vi "HeatFlow Results File Init.vi"(8 "error in":errorcluster, 9 "HeatFlow Res Cfg":T1, 11 "Log File Base Path":path) -> (0 "error out":errorcluster, 1 "Log File Name":string, 3 "Refnum out":refnum<k34>)   [LabVIEW 2019, in "Logging.lvlib"]
uses:
  Logging.lvlib
  HeatFlow Results States.ctl
  HeatFlow Res Cfg.ctl
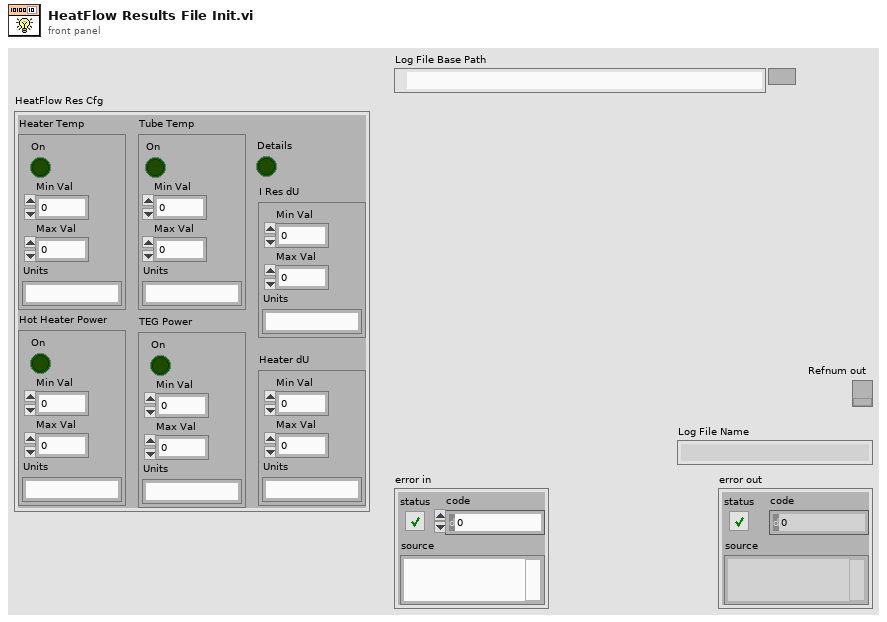
[diagram p1: front panel]
types:
  T1 = typedef "Logging.lvlib/HeatFlow Res Cfg.ctl" = cluster{"Heater Temp":cluster{"On":bool, "Min Val":dbl, "Max Val":dbl, "Units":string}, "Tube Temp":cluster{"On":bool, "Min Val":dbl, "Max Val":dbl, "Units":string}, "Hot Heater Power":cluster{"On":bool, "Min Val":dbl, "Max Val":dbl, "Units":string}, "TEG Power":cluster{"On":bool, "Min Val":dbl, "Max Val":dbl, "Units":string}, "Details":bool, "Heater dU":cluster{"Min Val":dbl, "Max Val":dbl, "Units":string}, "I Res dU":cluster{"Min Val":dbl, "Max Val":dbl, "Units":string}}
  T2 = typedef "Logging.lvlib/HeatFlow Results States.ctl" = enum16{"Start", "Timestamp", "Heater Temp", "Tube Temp", "Heater Power", "TEG Power", "Details", "End"}
  T3 = enum16{"open", "open or create", "create or replace", "create", "open (read-only)"}
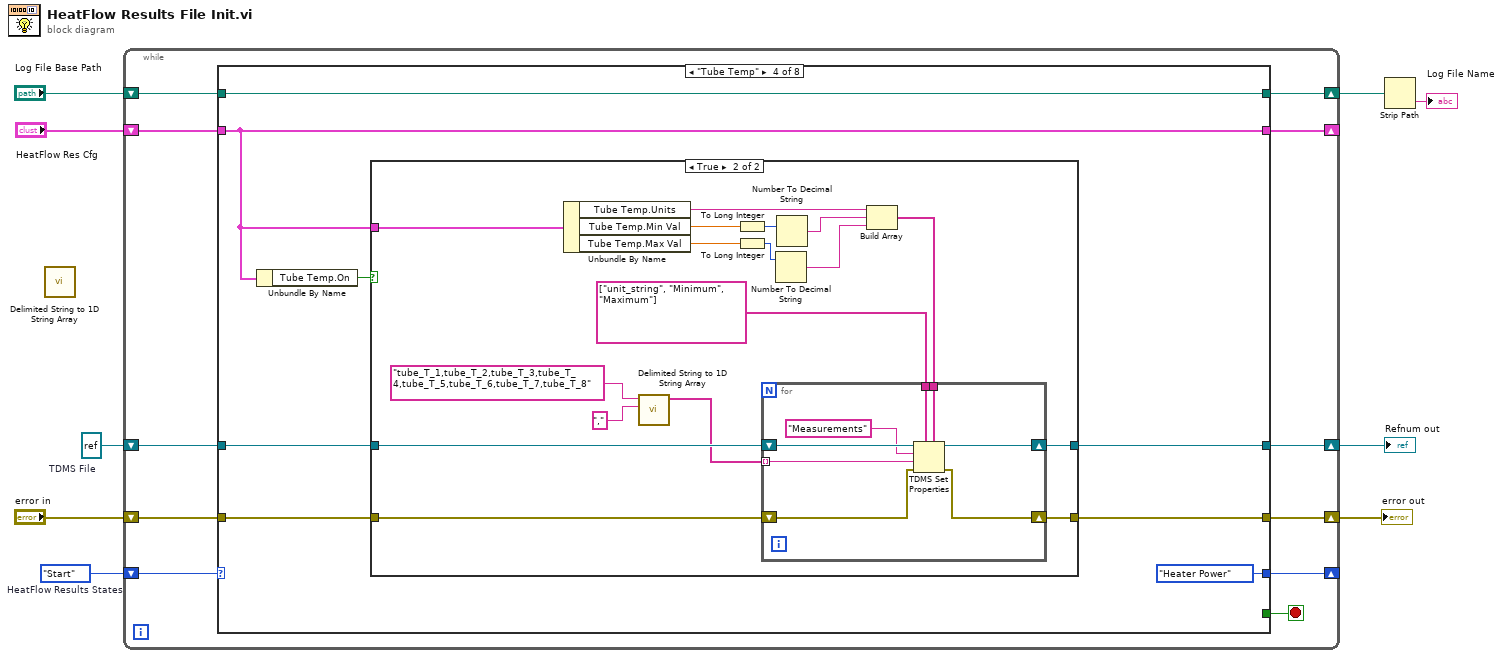
[diagram p0: block diagram]
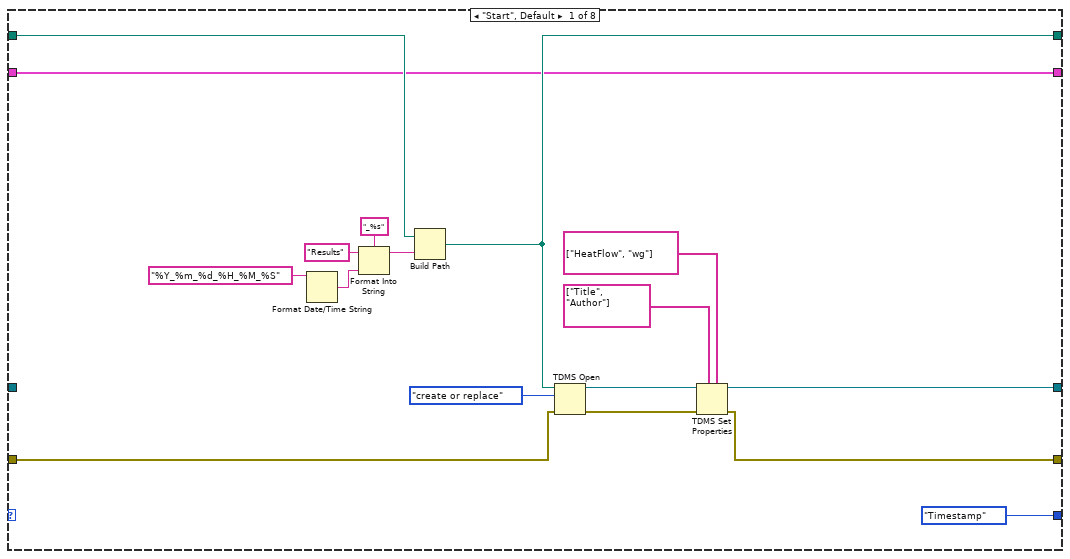
[diagram p2: hidden frame]
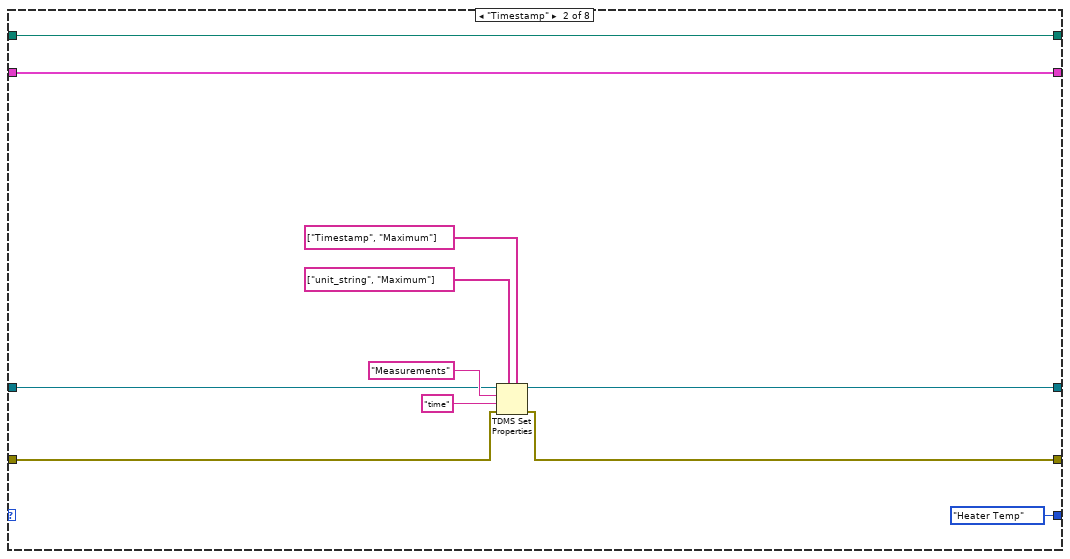
[diagram p3: hidden frame]
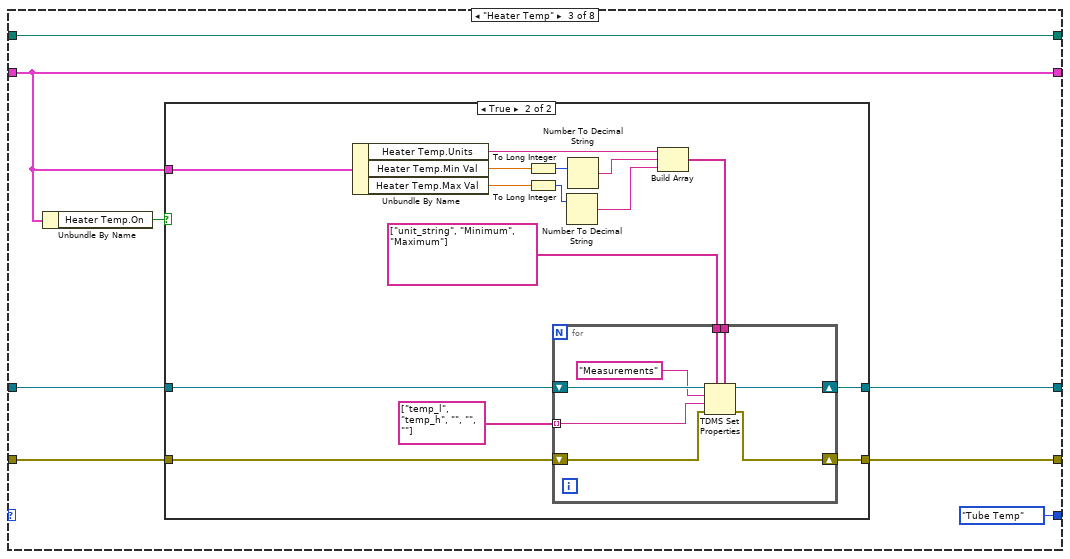
[diagram p4: hidden frame]
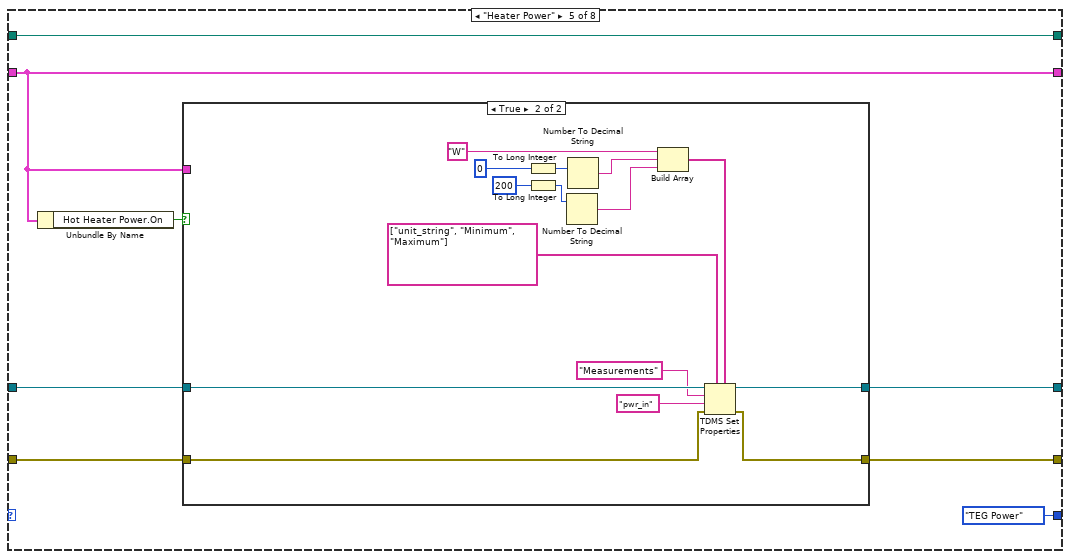
[diagram p7: hidden frame]
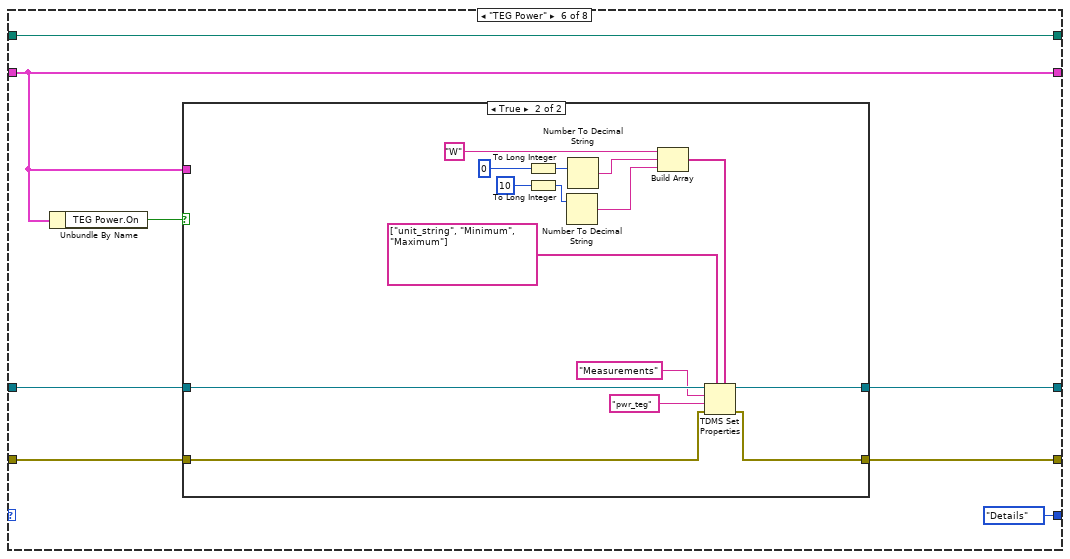
[diagram p9: hidden frame]
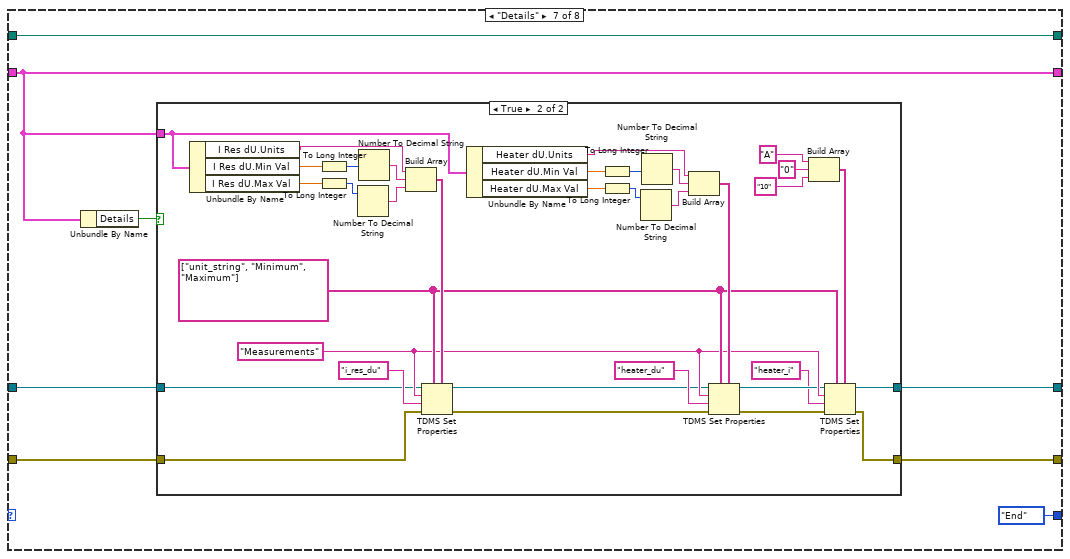
[diagram p11: hidden frame]
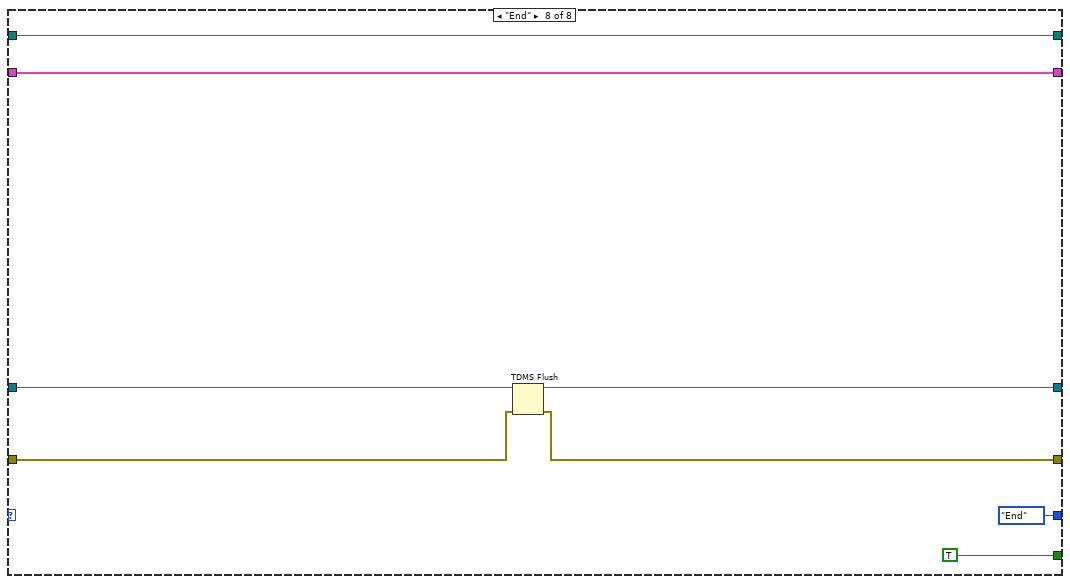
[diagram p13: hidden frame]
diagram:
  w2 = HeatFlow_Results_States."Start"  # HeatFlow Results States
  w8 = refnum<k34> refnum  # TDMS File
  n1 = call <vilib>:"Delimited String to 1D String Array.vi"() -> ()  [unwired: 11 in, 1 out]
  n2 = while {
    shift-right: [w10] -> _
    shift-left: w2 -> [w13]
    shift-right: [w17] -> w4
    shift-left: "Log File Base Path" -> [w20]
    shift-right: [w18] -> w7
    shift-left: "error in" -> [w19]
    shift-right: [w11] -> _
    shift-left: "HeatFlow Res Cfg" -> [w12]
    shift-right: [w15] -> w5
    shift-left: w8 -> [w16]
    stop <- w14 stop-if-true
    n3 = case shown="\"Tube Temp\"" w13 {
      tunnel: w20 -> [w31 w42 w56 w89 w124 w149 w173 w218]
      tunnel: w19 -> [w24 w41 w53 w86 w121 w146 w170 w214]
      tunnel: [w23 w40 w52 w85 w120 w145 w168 w213] -> w18
      tunnel: [w30 w42 w56 w89 w124 w149 w173 w218] -> w17
      tunnel: w16 -> [_ w44 w55 w88 w123 w148 w171 w216]
      tunnel: [w25 w43 w54 w87 w122 w147 w169 w215] -> w15
      tunnel: [_ _ _ _ _ _ _ TRUE] -> w14
      tunnel: w12 -> [w22 w39 w49 w82 w117 w142 w167 w212]
      tunnel: [w22 w39 w49 w82 w117 w142 w167 w212] -> w11
      tunnel: [HeatFlow_Results_States."Timestamp" ("Results") HeatFlow_Results_States."Heater Temp" ("Results") HeatFlow_Results_States."Tube Temp" ("Results") HeatFlow_Results_States."Heater Power" ("Results") HeatFlow_Results_States."TEG Power" ("Results") HeatFlow_Results_States."Details" ("Results") HeatFlow_Results_States."End" ("Results") HeatFlow_Results_States."End" ("Results")] -> w10
      frame "Start", Default {
        n4 = Format Date/Time String(time format string (%c)="%Y_%m_%d_%H_%M_%S") -> (date/time string=w37:string)  [unwired: 2 in]
        n5 = Format Into String(format string="_%s", initial string="Results", w37) -> (resulting string=w36:string)  [unwired: 1 in, 1 out]
        n6 = Build Path(base path=w31, name or relative path=w36) -> (appended path=w30:path)
        n7 = TDMS Open(8:w24, 10:T3."create or replace" ("operation (0:open)"), 11:w30) -> (0:w28:errorcluster, 3:w29:refnum<k34>)  [unwired: 4 in]
        n8 = TDMS Set Properties(5:string[] ["HeatFlow", "wg"] ("property names"), 7:string[] ["Title", "Author"] ("property names"), 8:w28, 11:w29) -> (0:w23:errorcluster, 3:w25:refnum<k34>)  [unwired: 2 in, 2 out]
      }
      frame "Timestamp" {
        n9 = TDMS Set Properties(5:string[] ["Timestamp", "Maximum"] ("property names"), 7:string[] ["unit_string", "Maximum"] ("property names"), 8:w41, 9:"time" ("channel name"), 10:"Measurements" ("group name in (Untitled)"), 11:w44) -> (0:w40:errorcluster, 3:w43:refnum<k34>)  [unwired: 2 out]
      }
      frame "Heater Temp" {
        n10 = Unbundle By Name(w49) -> ("Heater Temp.On"=w51:bool)
        n11 = case shown="True" w51 {
          tunnel: w55 -> [w58 w73]
          tunnel: [w58 w72] -> w54
          tunnel: w53 -> [w57 w71]
          tunnel: [w57 w70] -> w52
          tunnel: w49 -> [_ w62]
          frame False {
          }
          frame True {
            n12 = Unbundle By Name(w62) -> ("Heater Temp.Units"=w61:string, "Heater Temp.Min Val"=w60:dbl, "Heater Temp.Max Val"=w59:dbl)
            n13 = To Long Integer(number=w60) -> (32bit integer=w66:i32)
            n14 = To Long Integer(number=w59) -> (32bit integer=w65:i32)
            n15 = Number To Decimal String(number=w65) -> (decimal integer string=w63:string)  [unwired: 1 in]
            n16 = Number To Decimal String(number=w66) -> (decimal integer string=w64:string)  [unwired: 1 in]
            n17 = Build Array(w61, w64, w63) -> (w67:string[])
            n18 = for {
              shift-right: [w80] -> w72
              shift-left: w73 -> [w81]
              shift-right: [w77] -> w70
              shift-left: w71 -> [w78]
              tunnel: string[] ["temp_l", "temp_h", "", "", ""] -> [w76] mode=indexing
              tunnel: string[] ["unit_string", "Minimum", "Maximum"] ("property names") -> [w75]
              tunnel: w67 -> [w74]
              n19 = TDMS Set Properties(5:w74, 7:w75, 8:w78, 9:w76, 10:"Measurements" ("group name in (Untitled)"), 11:w81) -> (0:w77:errorcluster, 3:w80:refnum<k34>)  [unwired: 2 out]
            }
          }
        }
      }
      frame "Tube Temp" {
        n20 = Unbundle By Name(w82) -> ("Tube Temp.On"=w84:bool)
        n21 = case shown="True" w84 {
          tunnel: w88 -> [w91 w108]
          tunnel: [w91 w107] -> w87
          tunnel: w86 -> [w90 w106]
          tunnel: [w90 w105] -> w85
          tunnel: w82 -> [_ w95]
          frame False {
          }
          frame True {
            n22 = Unbundle By Name(w95) -> ("Tube Temp.Units"=w94:string, "Tube Temp.Min Val"=w93:dbl, "Tube Temp.Max Val"=w92:dbl)
            n23 = call <vilib>:"Delimited String to 1D String Array.vi"("delimiter"=",", "delimited string"="tube_T_1,tube_T_2,tube_T_3,tube_T_4,tube_T_5,tube_T_6,tube_T_7,tube_T_8" ("name to assign")) -> ("string array"=w97:string[])  [unwired: 9 in]
            n24 = To Long Integer(number=w93) -> (32bit integer=w102:i32)
            n25 = To Long Integer(number=w92) -> (32bit integer=w101:i32)
            n26 = Number To Decimal String(number=w101) -> (decimal integer string=w99:string)  [unwired: 1 in]
            n27 = Number To Decimal String(number=w102) -> (decimal integer string=w100:string)  [unwired: 1 in]
            n28 = Build Array(w94, w100, w99) -> (w103:string[])
            n29 = for {
              shift-right: [w115] -> w107
              shift-left: w108 -> [w116]
              shift-right: [w112] -> w105
              shift-left: w106 -> [w113]
              tunnel: w97 -> [w111] mode=indexing
              tunnel: string[] ["unit_string", "Minimum", "Maximum"] ("property names") -> [w110]
              tunnel: w103 -> [w109]
              n30 = TDMS Set Properties(5:w109, 7:w110, 8:w113, 9:w111, 10:"Measurements" ("group name in (Untitled)"), 11:w116) -> (0:w112:errorcluster, 3:w115:refnum<k34>)  [unwired: 2 out]
            }
          }
        }
      }
      frame "Heater Power" {
        n31 = Unbundle By Name(w117) -> ("Hot Heater Power.On"=w119:bool)
        n32 = case shown="True" w119 {
          tunnel: w123 -> [w126 w141]
          tunnel: [w126 w140] -> w122
          tunnel: w121 -> [w125 w139]
          tunnel: [w125 w138] -> w120
          tunnel: w117 -> [_ _]
          frame False {
          }
          frame True {
            n33 = To Long Integer(number=0) -> (32bit integer=w135:i32)
            n34 = To Long Integer(number=200) -> (32bit integer=w134:i32)
            n35 = Number To Decimal String(number=w134) -> (decimal integer string=w132:string)  [unwired: 1 in]
            n36 = Number To Decimal String(number=w135) -> (decimal integer string=w133:string)  [unwired: 1 in]
            n37 = Build Array("W" ("element"), w133, w132) -> (w136:string[])
            n38 = TDMS Set Properties(5:w136, 7:string[] ["unit_string", "Minimum", "Maximum"] ("property names"), 8:w139, 9:"pwr_in" ("channel name"), 10:"Measurements" ("group name in (Untitled)"), 11:w141) -> (0:w138:errorcluster, 3:w140:refnum<k34>)  [unwired: 2 out]
          }
        }
      }
      frame "TEG Power" {
        n39 = Unbundle By Name(w142) -> ("TEG Power.On"=w144:bool)
        n40 = case shown="True" w144 {
          tunnel: w148 -> [w151 w166]
          tunnel: [w151 w165] -> w147
          tunnel: w146 -> [w150 w164]
          tunnel: [w150 w163] -> w145
          tunnel: w142 -> [_ _]
          frame False {
          }
          frame True {
            n41 = To Long Integer(number=0) -> (32bit integer=w160:i32)
            n42 = To Long Integer(number=10) -> (32bit integer=w159:i32)
            n43 = Number To Decimal String(number=w159) -> (decimal integer string=w157:string)  [unwired: 1 in]
            n44 = Number To Decimal String(number=w160) -> (decimal integer string=w158:string)  [unwired: 1 in]
            n45 = Build Array("W" ("element"), w158, w157) -> (w161:string[])
            n46 = TDMS Set Properties(5:w161, 7:string[] ["unit_string", "Minimum", "Maximum"] ("property names"), 8:w164, 9:"pwr_teg" ("channel name"), 10:"Measurements" ("group name in (Untitled)"), 11:w166) -> (0:w163:errorcluster, 3:w165:refnum<k34>)  [unwired: 2 out]
          }
        }
      }
      frame "Details" {
        n47 = Unbundle By Name(w167) -> ("Details"=w172:bool)
        n48 = case shown="True" w172 {
          tunnel: w171 -> [w176 w187]
          tunnel: [w176 w184] -> w169
          tunnel: w170 -> [w175 w182]
          tunnel: [w175 w179] -> w168
          tunnel: w167 -> [_ w197]
          frame False {
          }
          frame True {
            w192 = "Measurements" ("group name in (Untitled)")
            w194 = string[] ["unit_string", "Minimum", "Maximum"] ("property names")
            n49 = Unbundle By Name(w197) -> ("I Res dU.Units"=w178:string, "I Res dU.Min Val"=w206:dbl, "I Res dU.Max Val"=w205:dbl)
            n50 = To Long Integer(number=w206) -> (32bit integer=w210:i32)
            n51 = To Long Integer(number=w205) -> (32bit integer=w209:i32)
            n52 = Number To Decimal String(number=w209) -> (decimal integer string=w207:string)  [unwired: 1 in]
            n53 = Number To Decimal String(number=w210) -> (decimal integer string=w208:string)  [unwired: 1 in]
            n54 = Build Array(w178, w208, w207) -> (w203:string[])
            n55 = TDMS Set Properties(5:w203, 7:w194, 8:w182, 9:"i_res_du", 10:w192, 11:w187) -> (0:w181:errorcluster, 3:w186:refnum<k34>)  [unwired: 2 out]
            n56 = Unbundle By Name(w197) -> ("Heater dU.Units"=w177:string, "Heater dU.Min Val"=w199:dbl, "Heater dU.Max Val"=w198:dbl)
            n57 = To Long Integer(number=w199) -> (32bit integer=w202:i32)
            n58 = To Long Integer(number=w198) -> (32bit integer=w201:i32)
            n59 = Number To Decimal String(number=w201) -> (decimal integer string=w196:string)  [unwired: 1 in]
            n60 = Number To Decimal String(number=w202) -> (decimal integer string=w200:string)  [unwired: 1 in]
            n61 = Build Array(w177, w200, w196) -> (w195:string[])
            n62 = TDMS Set Properties(5:w195, 7:w194, 8:w181, 9:"heater_du", 10:w192, 11:w186) -> (0:w180:errorcluster, 3:w185:refnum<k34>)  [unwired: 2 out]
            n63 = Build Array("A" ("element"), "0" ("element"), "10" ("element")) -> (w188:string[])
            n64 = TDMS Set Properties(5:w188, 7:w194, 8:w180, 9:"heater_i", 10:w192, 11:w185) -> (0:w179:errorcluster, 3:w184:refnum<k34>)  [unwired: 2 out]
          }
        }
      }
      frame "End" {
        n65 = TDMS Flush(4:w214, 7:w216) -> (0:w213:errorcluster, 3:w215:refnum<k34>)
      }
    }
  }
  "error out" <- w7
  "Refnum out" <- w5
  n66 = Strip Path(path=w4) -> (name=→"Log File Name":string)  [unwired: 1 out]
